vi "_042.vi"() -> ()   [LabVIEW 2024]
panel:
  in  "Boolean":bool
  out "Process":string
  in  "Enum":T1(ring)
  out "o/p":dbl
  in  "B":dbl
  in  "A":dbl
  # "Basic State Machine :"
  # "without using Event structure"
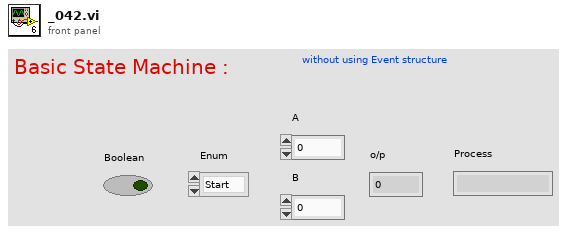
[diagram p1: front panel]
types:
  T1 = enum16{"Start", "Add", "Sub", "Mul", "Div", "Stop"}
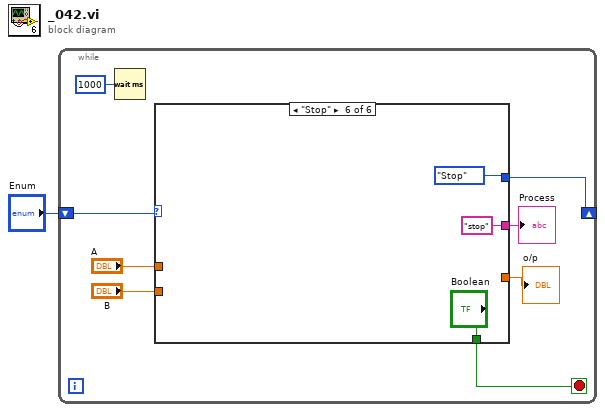
[diagram p0: block diagram]
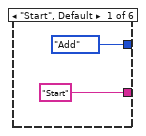
[diagram p2: hidden frame]
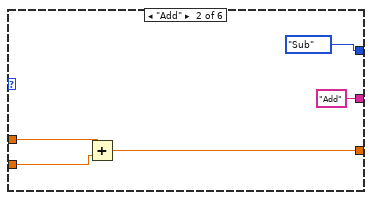
[diagram p3: hidden frame]
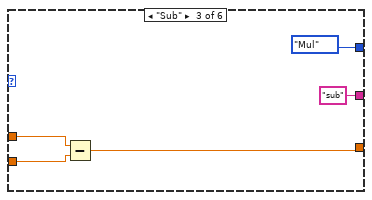
[diagram p4: hidden frame]
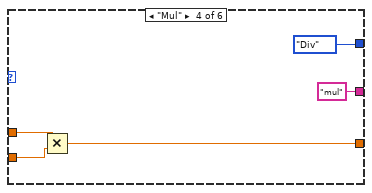
[diagram p5: hidden frame]
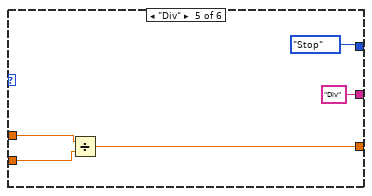
[diagram p6: hidden frame]
diagram:
  n1 = while {
    shift-right: [w6] -> _
    shift-left: "Enum" -> [w9]
    stop <- w7 stop-if-true
    n2 = Wait (ms)(milliseconds to wait=u32 1000) -> ()  [unwired: 1 out]
    n3 = case shown="\"Stop\"" w9 {
      tunnel: ["Start" "Add" "sub" "mul" "Div" "stop"] -> w8
      tunnel: [_ _ _ _ _ "Boolean"] -> w7
      tunnel: [T1."Add" ("Enum 2") T1."Sub" ("Enum 2") T1."Mul" ("Enum 2") T1."Div" ("Enum 2") T1."Stop" ("Enum 2") T1."Stop" ("Enum 2")] -> w6
      tunnel: "A" -> [_ w15 w20 w25 w30 _]
      tunnel: "B" -> [_ w14 w19 w24 w29 _]
      tunnel: [_ w13 w18 w23 w28 _] -> w3
      frame "Start", Default {
      }
      frame "Add" {
        n4 = Add(x=w15, y=w14) -> (x+y=w13:dbl)
      }
      frame "Sub" {
        n5 = Subtract(x=w20, y=w19) -> (x-y=w18:dbl)
      }
      frame "Mul" {
        n6 = Multiply(x=w25, y=w24) -> (x*y=w23:dbl)
      }
      frame "Div" {
        n7 = Divide(x=w30, y=w29) -> (x/y=w28:dbl)
      }
      frame "Stop" {
      }
    }
    "Process" <- w8
    "o/p" <- w3
  }
